vi "Configure Trigger.vi"(0 "VISA resource name":refnum<visa-resource-name>, 1 "Trigger Transient Source (0:Software)":u16(ring) items=["Software", "External", "Immediate"], 5 "Trigger Delay (0 Sec)":dbl, 7 "Trigger Synchronize Source (0:Immediate)":u16(ring) items=["Immediate", "Phase"], 9 "Trigger Synchronize Phase (0°)":dbl, 11 "error in (no error)":errorcluster, 12 "Trigger Acquire Source (0:Software)":u16(ring) items=["Software", "External", "TTL Trigger"]) -> (4 "VISA resource name out":refnum<visa-resource-name>, 15 "error out":errorcluster)   [LabVIEW 2010, in "California Instruments iX Series.lvlib"]
doc: "Configures the trigger setup such as trigger sources, delay and phase."
uses:
  <instrlib>/California Instruments iX Series/California Instruments iX Series.lvlib
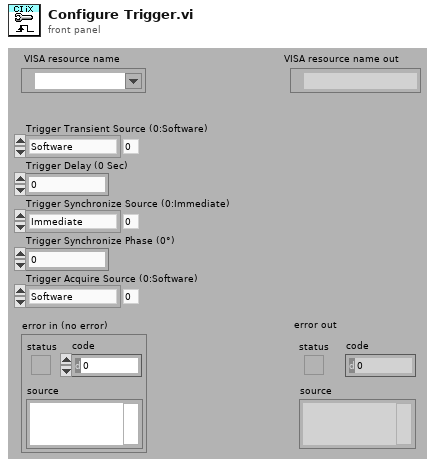
[diagram p1: front panel]
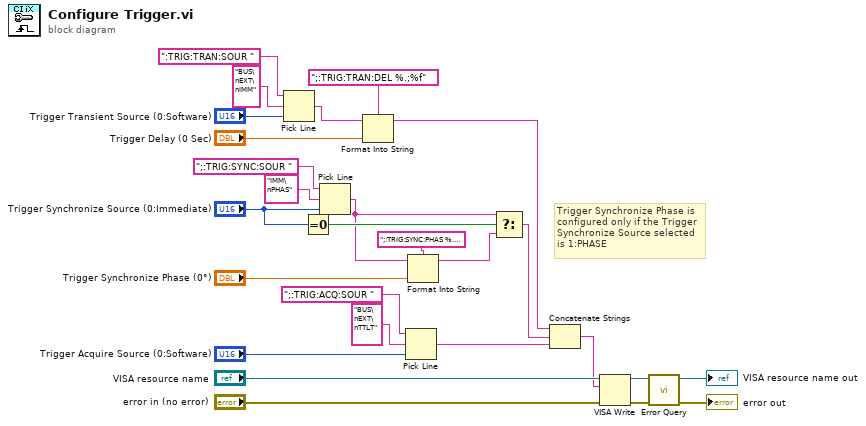
[diagram p0: block diagram]
diagram:
  # "Trigger Synchronize Phase is configured only if the Trigger Synchronize Source selected is 1:PHASE"
  n1 = Pick Line(string ("")=":TRIG:TRAN:SOUR ", multi-line string="BUS\nEXT\nIMM", line index="Trigger Transient Source (0:Software)") -> (output string=w17:string)
  n2 = Equal To 0?(x="Trigger Synchronize Source (0:Immediate)") -> (x = 0?=w9:bool)
  n3 = Pick Line(string ("")=";:TRIG:SYNC:SOUR ", multi-line string="IMM\nPHAS", line index="Trigger Synchronize Source (0:Immediate)") -> (output string=w8:string)
  n4 = Format Into String(format string=";:TRIG:TRAN:DEL %.;%f", initial string=w17, "Trigger Delay (0 Sec)") -> (resulting string=w13:string)  [unwired: 1 in, 1 out]
  n5 = Pick Line(string ("")=";:TRIG:ACQ:SOUR ", multi-line string="BUS\nEXT\nTTLT", line index="Trigger Acquire Source (0:Software)") -> (output string=w2:string)
  n6 = Format Into String(format string=";:TRIG:SYNC:PHAS %.;%f", initial string=w8, "Trigger Synchronize Phase (0°)") -> (resulting string=w6:string)  [unwired: 1 in, 1 out]
  n7 = Select(t=w8, s=w9, f=w6) -> (s? t:f=w7:string)
  n8 = Concatenate Strings(w13, w7, w2) -> (w1:string)
  n9 = VISA Write(VISA resource name="VISA resource name", write buffer=w1, error in (no error)="error in (no error)") -> (VISA resource name out=w25:refnum<visa-resource-name>, error out=w24:errorcluster)  [unwired: 1 out]
  n10 = call <instrlib>:"Error Query.vi"("error in (no error)"=w24, "VISA resource name"=w25) -> ("error out"=→"error out":errorcluster, "VISA resource name out"=→"VISA resource name out":refnum<visa-resource-name>)  [unwired: 6 in, 2 out]
